vi "Reset.vi"(8 "error in (no error)":errorcluster, 11 "senseHatDisplay in":refnum<class "RPI.SenseHat.Display.lvclass">) -> (0 "error out":errorcluster, 3 "senseHatDisplay out":refnum<class "RPI.SenseHat.Display.lvclass">)   [LabVIEW 2020, in "RPI.SenseHat.Display.lvlib" / "RPI.SenseHat.Display.lvclass"]
doc: "Resets the screen with the start-up rainbow colors.\n\nNote: Requires a call to Update to affect the physical screen."
uses:
  RPI.SenseHat.Display.lvclass
  Pixel/Pixel.lvclass
  Image/Image.lvclass
  Color/Color.lvclass
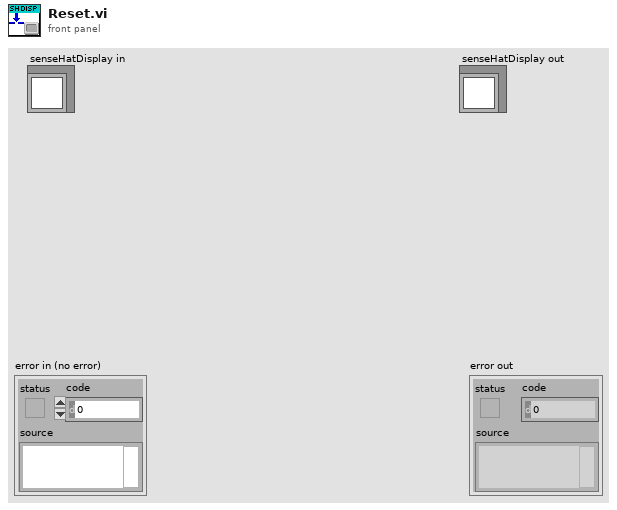
[diagram p1: front panel]
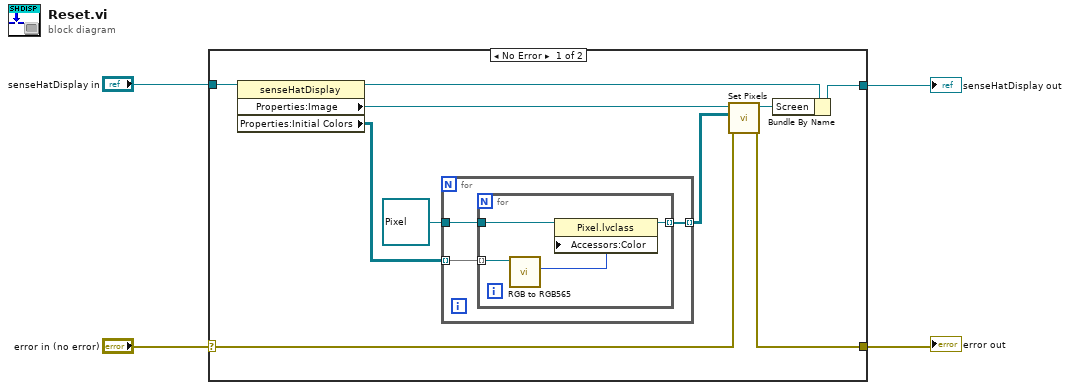
[diagram p0: block diagram]
diagram:
  n1 = case shown="No Error" "error in (no error)" {
    selector: "error in (no error)" -> [w8 w23]
    tunnel: [w7 w23] -> w3
    tunnel: [w14 w22] -> w1
    tunnel: "senseHatDisplay in" -> [w12 w22]
    frame No Error {
      n2 = property class="senseHatDisplay"(reference=w12) -> (reference out=w13:refnum<class "RPI.SenseHat.Display.lvclass">, "Properties:Image"=w5:refnum<class "Image.lvclass">, "Properties:Initial Colors"=w6:refnum<class "Color.lvclass">[][])  [unwired: 1 in, 1 out]
      n3 = for {
        tunnel: w6 -> [w17] mode=indexing
        tunnel: [w16] -> w9 mode=indexing
        tunnel: refnum<class "Pixel.lvclass"> refnum ("Pixel.lvclass") -> [w15]
        n4 = for {
          tunnel: w17 -> [w19] mode=indexing
          tunnel: [w21] -> w16 mode=indexing
          tunnel: w15 -> [w20]
          n5 = call "RGB to RGB565.vi"("Color in"=w19) -> ("Color"=w18:u16)  [unwired: 8 in, 2 out]
          n6 = property class="Pixel.lvclass"(reference=w20, "Accessors:Color"=w18) -> (reference out=w21:refnum<class "Pixel.lvclass">)  [unwired: 1 in, 1 out]
        }
      }
      n7 = call "Set Pixels.vi"("error in (no error)"=w8, "Pixels"=w9, "Image in"=w5) -> ("error out"=w7:errorcluster, "Image out"=w10:refnum<class "Image.lvclass">)  [unwired: 7 in]
      n8 = Bundle By Name(cluster=w13, "Screen"=w10) -> (w14:refnum<class "RPI.SenseHat.Display.lvclass">)
    }
    frame Error {
    }
  }
  "error out" <- w3
  "senseHatDisplay out" <- w1
